vi "Voltage_Input-Clear_initial_data.vi"() -> ()   [LabVIEW 2018]
doc: "This example demonstrates how to continuously acquire buffered voltage measurements using a DAQmx device.\n\nFor instructions on how to connect your signals to the DAQ device, refer to your device documentation."
uses:
  <vilib>/Utility/error.llb/DialogType.ctl
  <vilib>/DAQmx/read.llb/DAQmx Read (Analog 1D DBL NChan 1Samp).vi
  <vilib>/DAQmx/read.llb/DAQmx Read (Analog 1D Wfm NChan NSamp).vi
  <vilib>/DAQmx/create/channels.llb/DAQmx Create Channel (AI-Voltage-Basic).vi
  <vilib>/DAQmx/configure/timing.llb/DAQmx Timing (Sample Clock).vi
  <vilib>/DAQmx/miscellaneous.llb/DAQmx Fill In Error Info.vi
  <resource>/objmgr/daqmx.rc
panel:
  out "data":dbl[](array[numeric]) format="%0.2f"
  out "Waveform Chart 7":waveform(dbl)(graph)={"t0"=timestamp(7.03905963988022 s since 1904-01-01), "dt"=0.001, "Y"=array[1000 elements], "attributes"=variant("NI_ChannelName"=variant(string "cDAQ1Mod1/ai0"), "NI_UnitDescription"=variant(string "Volts"))}
  out "Waveform Chart 6":waveform(dbl)(graph)
  out "Waveform Chart 5":waveform(dbl)(graph)
  out "Waveform Chart 3":waveform(dbl)(graph)
  in  "samples per channel":i32=1000
  in  "Stop 2":bool
  in  "name or relative path":string
  in  "Sample Rate":dbl=1000.0
  in  "Max Voltage":dbl=5.0
  in  "Min Voltage":dbl=-5.0
  out "Actual Sample Rate":dbl=1000.0 format="%0.2f"
  # "Volt Input"
  # "Channel 1"
  # "Channel 2"
  # "Channel 3"
  # "Channel 4"
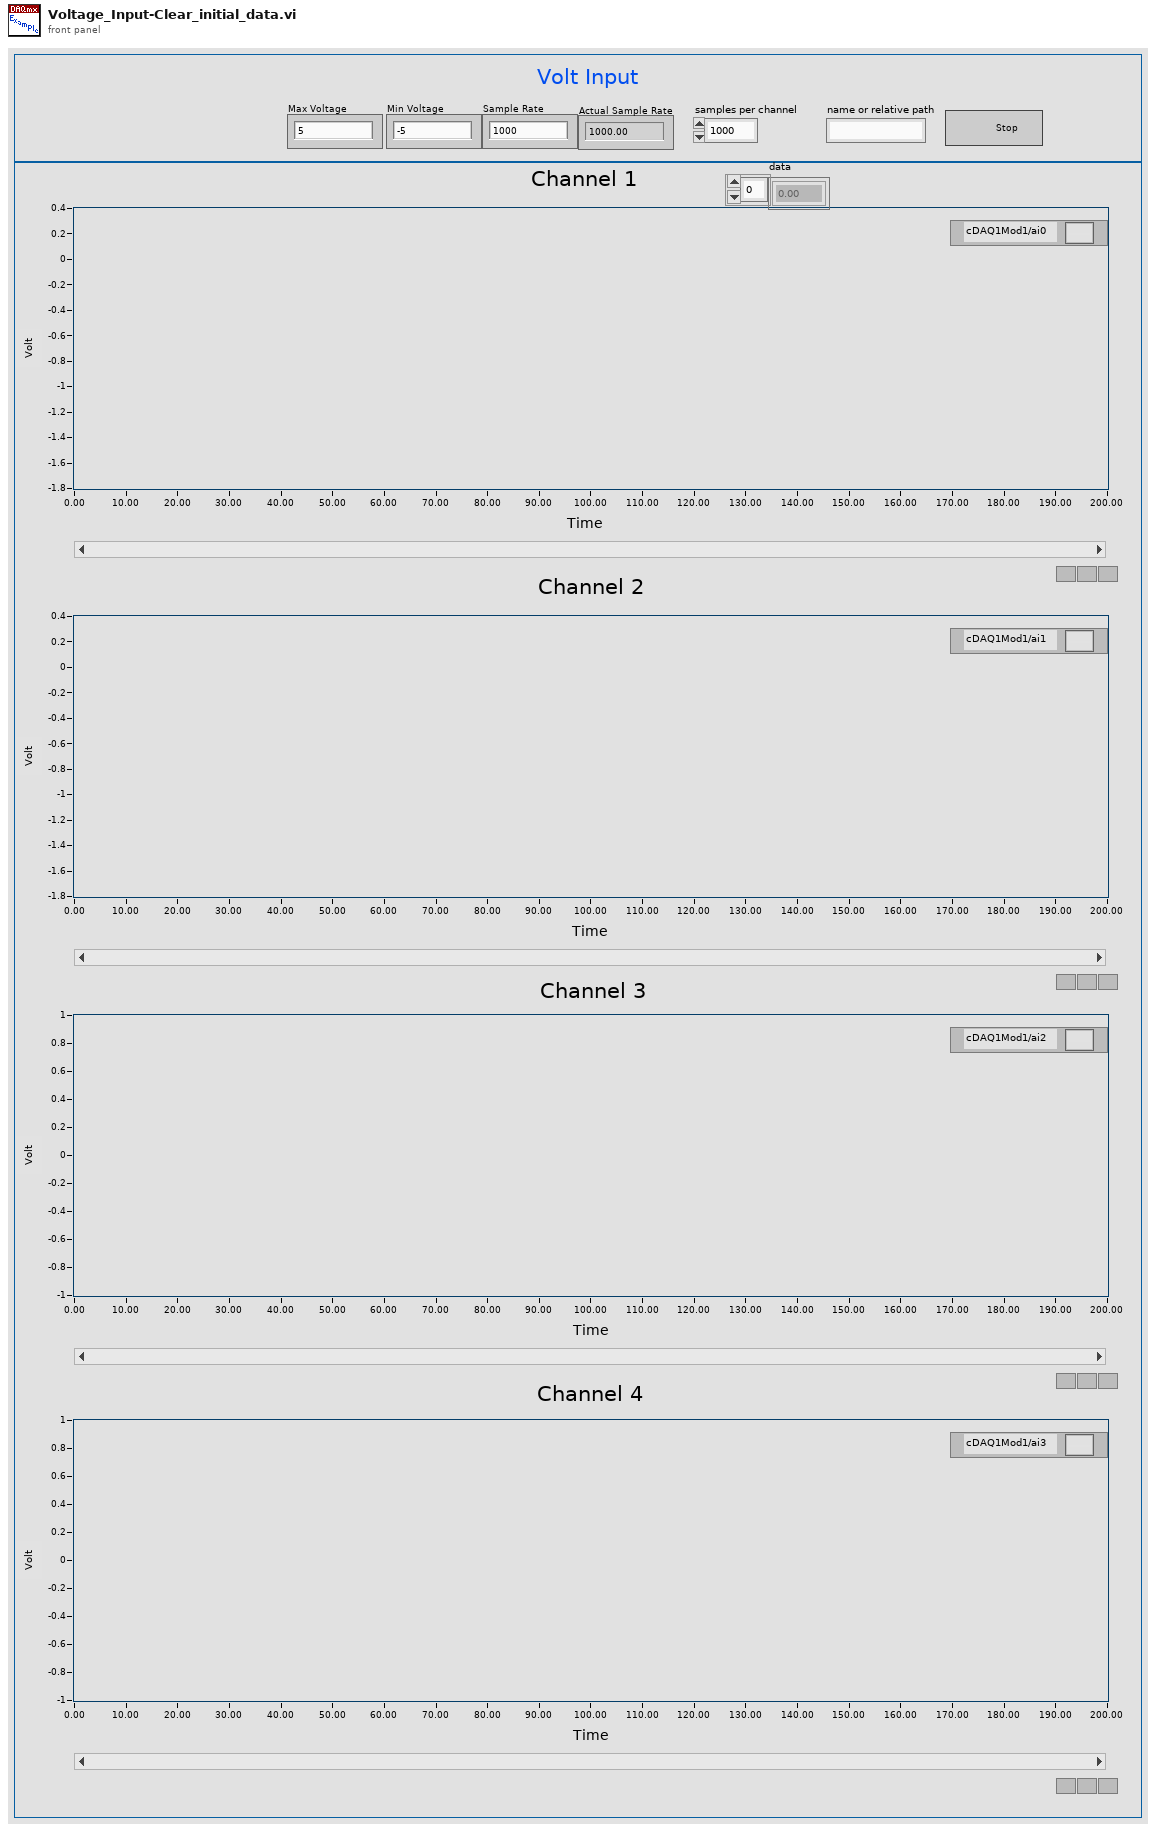
[diagram p1: front panel]
types:
  T1 = typedef "DialogType.ctl" = u16
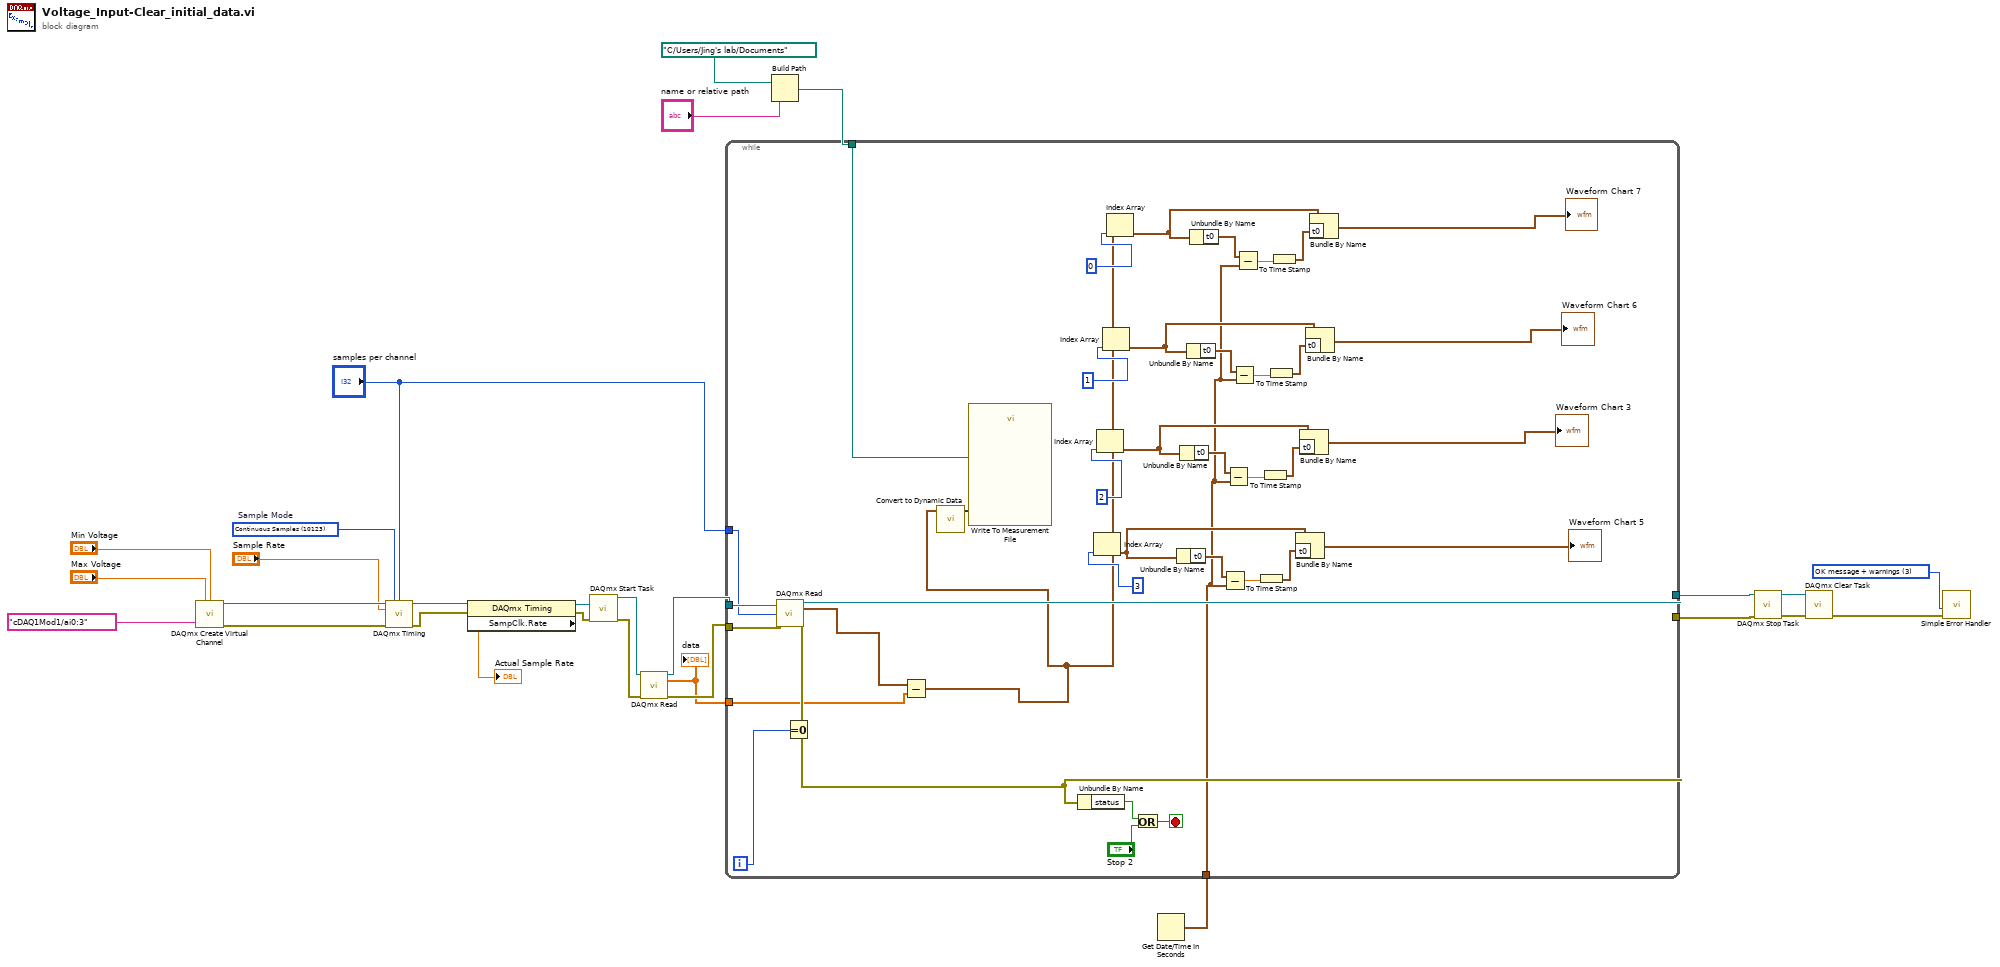
[diagram p0: block diagram]
diagram:
  w13 = T1 3 items=["no dialog", "OK message", "continue or stop message", "OK message + warnings", "continue/stop + warnings"] ("type of dialog (OK msg:1)")
  w26 = 10123 items=["Finite Samples"=10178, "Continuous Samples"=10123, "Hardware Timed Single Point"=12522]  # Sample Mode
  n1 = call-poly <vilib>:"DAQmx Create Virtual Channel.vi"("maximum value"="Max Voltage", "minimum value"="Min Voltage", "physical channels"=tag "cDAQ1Mod1/ai0:3" ("Physical Channel")) -> ("task out"=w24:refnum<k21>, "error out"=w25:errorcluster)  [unwired: 11 in]
  n2 = call-poly <vilib>:"DAQmx Timing.vi"("task/channels in"=w24, "sample mode"=w26, "samples per channel"="samples per channel", "rate"="Sample Rate", "error in"=w25) -> ("task out"=w28:refnum<k21>, "error out"=w27:errorcluster)  [unwired: 9 in]
  n3 = property class="DAQmx Timing"(reference=w28, error in=w27) -> (reference out=w9:refnum<k21>, error out=w10:errorcluster, "SampClk.Rate"=→"Actual Sample Rate":dbl)
  n4 = call <vilib>:"DAQmx Start Task.vi"("task/channels in"=w9, "error in"=w10) -> ("task out"=w5:refnum<k21>, "error out"=w4:errorcluster)  [unwired: 12 in]
  n5 = call-poly <vilib>:"DAQmx Read.vi"("task/channels in"=w5, "error in"=w4) -> ("task out"=w3:refnum<k21>, "data"=w1:dbl[], "error out"=w2:errorcluster)  [unwired: 11 in]
  "data" <- w1
  n6 = Build Path(base path=path "C:/Users/Jing's lab/Documents", name or relative path="name or relative path") -> (appended path=w8:path)
  n7 = Get Date/Time In Seconds() -> (seconds since 1Jan1904=w6:timestamp)
  n8 = while {
    tunnel: w3 -> [w67]
    tunnel: w2 -> [w66]
    tunnel: [w65] -> w17
    tunnel: [w64] -> w16
    tunnel: w8 -> [w61]
    tunnel: "samples per channel" -> [w59]
    tunnel: w6 -> [w34]
    tunnel: w1 -> [w31]
    i -> [w33]
    stop <- w62 stop-if-true
    n9 = call-poly <vilib>:"DAQmx Read.vi"("task/channels in"=w67, "number of samples per channel"=w59, "error in"=w66) -> ("task out"=w65:refnum<k21>, "data"=w30:waveform(dbl)[], "error out"=w64:errorcluster)  [unwired: 10 in]
    n10 = Equal To 0?(x=w33) -> ()  [unwired: 1 out]
    n11 = Subtract(x=w30, y=w31) -> (x-y=w29:waveform(dbl)[])
    n12 = call "Convert to Dynamic Data"("Array"=w29) -> ("Dynamic Data Type"=w32:dynamicdata)  [unwired: 3 in]
    n13 = call "Write To Measurement File"("Signals"=w32, "Filename"=w61) -> ()  [unwired: 15 in, 3 out]
    n14 = Unbundle By Name(w64) -> ("status"=w63:bool)
    n15 = Index Array(array=w29, index=3 ("Channel 4")) -> (element=w55:waveform(dbl))
    n16 = Index Array(array=w29, index=2 ("Channel 3")) -> (element=w51:waveform(dbl))
    n17 = Index Array(array=w29, index=1 ("Channel 2")) -> (element=w42:waveform(dbl))
    n18 = Index Array(array=w29, index=0 ("Channel 1")) -> (element=w39:waveform(dbl))
    n19 = Or(x=w63, y="Stop 2") -> (x .or. y?=w62:bool)
    n20 = Unbundle By Name(w55) -> ("t0"=w58:timestamp)
    n21 = Unbundle By Name(w51) -> ("t0"=w48:timestamp)
    n22 = Unbundle By Name(w42) -> ("t0"=w45:timestamp)
    n23 = Unbundle By Name(w39) -> ("t0"=w36:timestamp)
    n24 = Subtract(x=w58, y=w34) -> (x-y=w57:dbl)
    n25 = Subtract(x=w48, y=w34) -> (x-y=w49:dbl)
    n26 = Subtract(x=w45, y=w34) -> (x-y=w44:dbl)
    n27 = Subtract(x=w36, y=w34) -> (x-y=w37:dbl)
    n28 = To Time Stamp(1:w57) -> (0:w56:timestamp)
    n29 = To Time Stamp(1:w49) -> (0:w50:timestamp)
    n30 = To Time Stamp(1:w44) -> (0:w43:timestamp)
    n31 = To Time Stamp(1:w37) -> (0:w38:timestamp)
    n32 = Bundle By Name(cluster=w55, "t0"=w56) -> (→"Waveform Chart 5":waveform(dbl))
    n33 = Bundle By Name(cluster=w51, "t0"=w50) -> (→"Waveform Chart 3":waveform(dbl))
    n34 = Bundle By Name(cluster=w42, "t0"=w43) -> (→"Waveform Chart 6":waveform(dbl))
    n35 = Bundle By Name(cluster=w39, "t0"=w38) -> (→"Waveform Chart 7":waveform(dbl))
  }
  n36 = call <vilib>:"DAQmx Stop Task.vi"("task/channels in"=w17, "error in"=w16) -> ("task out"=w14:refnum<k21>, "error out"=w15:errorcluster)  [unwired: 12 in]
  n37 = call <vilib>:"DAQmx Clear Task.vi"("task in"=w14, "error in"=w15) -> ("error out"=w23:errorcluster)  [unwired: 13 in]
  n38 = call <vilib>:"Simple Error Handler.vi"("type of dialog (OK msg:1)"=w13, "error in (no error)"=w23) -> ()  [unwired: 3 in, 5 out]
